vi "JSON to Variant.vi"(7 "Variant Type":variant, 8 "error in (no error)":errorcluster, 10 "JSON Path (\"\"=Root)":string[](array[string]), 11 "JSON":string) -> (0 "error out":errorcluster, 3 "Variant out":variant)   [LabVIEW 2019, in "labview_json.lvlib"]
doc: "Imports a <b>JSON</b> string to a <b>Variant</b>. If <b>Variant Type</b> is not specified, this returns the native JSON data types. Specify the <b>JSON Path</b> to get a nested object key or array index.\nCreated by: Ryan Pacini"
uses:
  labview_json.lvlib
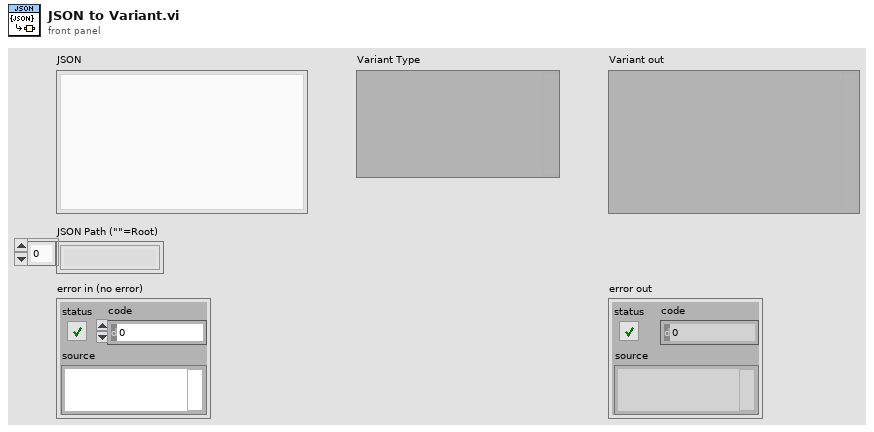
[diagram p1: front panel]
types:
  T1 = typedef "labview_json.lvlib/Value.ctl" = cluster{"Key":string, "Type":T2, "Value":variant}
  T2 = typedef "labview_json.lvlib/Value Type.ctl" = enum8{"NULL", "OBJECT", "ARRAY", "BOOL", "INT", "UINT", "FLOAT", "STRING"}
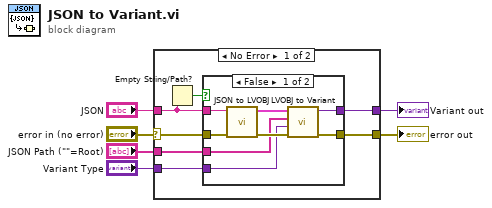
[diagram p0: block diagram]
diagram:
  n1 = case shown="No Error" "error in (no error)" {
    selector: "error in (no error)" -> [w13 w25]
    tunnel: [w12 w25] -> w5
    tunnel: "JSON" -> [w10 _]
    tunnel: [w11 w24] -> w3
    tunnel: "Variant Type" -> [w8 w24]
    tunnel: "JSON Path (\"\"=Root)" -> [w7 _]
    frame No Error {
      n2 = Empty String/Path?(string/path=w10) -> (empty?=w9:bool)
      n3 = case shown="False" w9 {
        tunnel: w13 -> [w21 w23]
        tunnel: w10 -> [w20 _]
        tunnel: [w19 w23] -> w12
        tunnel: [w17 w22] -> w11
        tunnel: w8 -> [w15 w22]
        tunnel: w7 -> [w14 _]
        frame False {
          n4 = call "JSON to LVOBJ.vi"("error in (no error)"=w21, "JSON"=w20) -> ("error out"=w16:errorcluster, "Root"=w18:T1)  [unwired: 8 in]
          n5 = call "LVOBJ to Variant.vi"("error in (no error)"=w16, "Variant Type"=w15, "JSON Path"=w14, "Root"=w18) -> ("error out"=w19:errorcluster, "Variant out"=w17:variant)  [unwired: 5 in, 1 out]
        }
        frame True {
        }
      }
    }
    frame Error {
    }
  }
  "error out" <- w5
  "Variant out" <- w3
